vi "LV86_Mirror.vi"(3 "Image":T1 {"Dialogs" format="%.0b"}) -> (1 "Image":T1 {"Dialogs" format="%.0b"})   [LabVIEW 2024]
doc: "This VI mirrors the input image (vertical symmetry). The image may be any type (binary, greyscale or RGB)."
uses:
  <userlib>/ImageProcessing/QTLIB_2595_LV86/QT_Image.ctl
panel:
  # "This VI mirrors the input image (vertical symmetry).  The image may be any \ntype (binary, greyscale or RGB)."
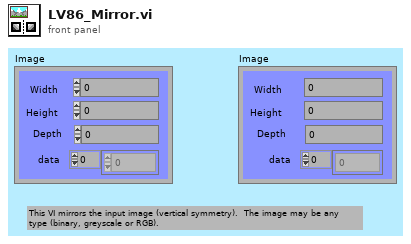
[diagram p1: front panel]
types:
  T1 = typedef "QT_Image.ctl" = cluster{"Width":i32, "Height":i32, "Depth":i32, "data":u8[], "Compressed data":u8[], "Color table":u32[], "Duration":i32, "Options":i32, "Timestamp":i32, "ID":i32, "Reserved":i32, "Dialogs":u32}
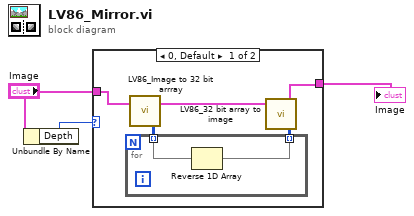
[diagram p0: block diagram]
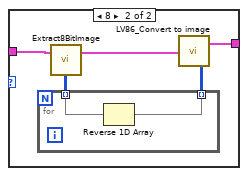
[diagram p2: hidden frame]
diagram:
  n1 = Unbundle By Name("Image") -> ("Depth"=w3:i32)
  n2 = case shown="0, Default" w3 {
    tunnel: "Image" -> [w8 w15]
    tunnel: [w6 w13] -> w1
    frame 0, Default {
      n3 = call <userlib>:"LV86_Image to 32 bit arrray.vi"("Image In"=w8) -> ("Intensity Graph"=w5:u32[][], "Image out"=w7:T1)  [unwired: 1 in]
      n4 = for {
        tunnel: w5 -> [w10] mode=indexing
        tunnel: [w9] -> w4 mode=indexing
        n5 = Reverse 1D Array(array=w10) -> (reversed array=w9:u32[])
      }
      n6 = call <userlib>:"LV86_32 bit array to image.vi"("Intensity Graph"=w4, "Image In"=w7) -> ("Image Out"=w6:T1)  [unwired: 1 in]
    }
    frame 8 {
      n7 = call <userlib>:"Extract8BitImage.vi"("Image in"=w15) -> ("Intensity Graph"=w12:u8[][], "Image out"=w14:T1)  [unwired: 1 in]
      n8 = for {
        tunnel: w12 -> [w17] mode=indexing
        tunnel: [w16] -> w11 mode=indexing
        n9 = Reverse 1D Array(array=w17) -> (reversed array=w16:u8[])
      }
      n10 = call <userlib>:"LV86_Convert to image.vi"("Intensity Graph"=w11, "Image In"=w14) -> ("Image Out"=w13:T1)  [unwired: 1 in]
    }
  }
  "Image" <- w1
